vi "Handle Vecto Message.vi"(8 "error in (no error)":errorcluster, 10 "TcpPayload":T1, 11 "Task in":refnum<class "Task.lvclass">) -> (0 "error out":errorcluster, 3 "Task out":refnum<class "Task.lvclass">)   [LabVIEW 2020, in "Volatus.lvlib" / "Task.lvclass"]
uses:
  Task.lvclass
  Task.lvclass/Task.ctl
  lv-vecto/Vecto/proto/TcpPayload/Data.ctl
  lv-vecto/Vecto/proto/TcpPayload/TcpPayload.lvlib
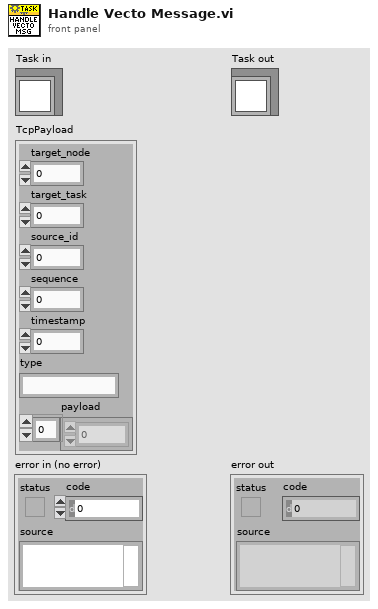
[diagram p1: front panel]
types:
  T1 = typedef "TcpPayload.lvlib/Data.ctl" = cluster{"target_node":u32, "target_task":u32, "source_id":u32, "sequence":u32, "timestamp":u64, "type":string, "payload":u8[]}
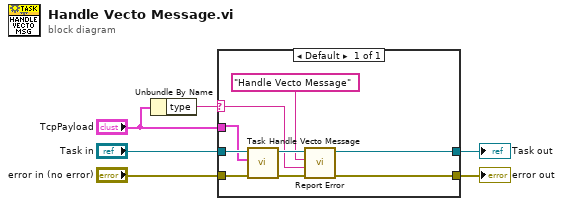
[diagram p0: block diagram]
diagram:
  n1 = Unbundle By Name("TcpPayload") -> ("type"=w4:string)
  n2 = case shown="Default" w4 {
    selector: w4 -> [w10]
    tunnel: "Task in" -> [w15]
    tunnel: "error in (no error)" -> [w14]
    tunnel: "TcpPayload" -> [w13]
    tunnel: [w8] -> w2
    tunnel: [w7] -> w1
    frame Default {
      n3 = call-dynamic "Task Handle Vecto Message.vi"("error in (no error)"=w14, "TcpPayload"=w13, "Task in"=w15) -> ("error out"=w12:errorcluster, "Task out"=w11:refnum<class "Task.lvclass">)  [unwired: 7 in]
      n4 = call "Report Error.vi"("error in (no error)"=w12, "Message"=w10, "Context"="Handle Vecto Message", "Task in"=w11) -> ("error out"=w8:errorcluster, "Task out"=w7:refnum<class "Task.lvclass">)  [unwired: 6 in]
    }
  }
  "error out" <- w2
  "Task out" <- w1
